vi "GitLab Mass Editor.vi"() -> ()   [LabVIEW 2020]
panel:
  in  "Edit Mode":enum16{"Add Section", "Remove Section"}(ring)
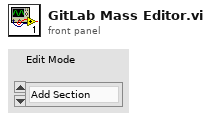
[diagram p1: front panel]
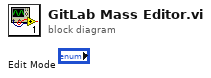
[diagram p0: block diagram]
diagram:
